vi "Handle Command.vi"(8 "error in (no error)":errorcluster, 9 "Data":variant, 10 "Command":string, 11 "VNA":refnum<class "VNA.lvclass">) -> (0 "error out":errorcluster, 1 "Processed Data":variant, 2 "Command":string, 3 "VNA out":refnum<class "VNA.lvclass">)   [LabVIEW 2016, in "VNA.lvclass"]
uses:
  VNA.lvclass
  VNA.lvclass/VNA.ctl
  <userlib>/LevyLab/Levylab Instruments/Instrument Types/VNA/Instrument.VNA.lvclass
  P:/users1/Dengyu/Agilent 87XX Series/Agilent 87XX Series.lvlib
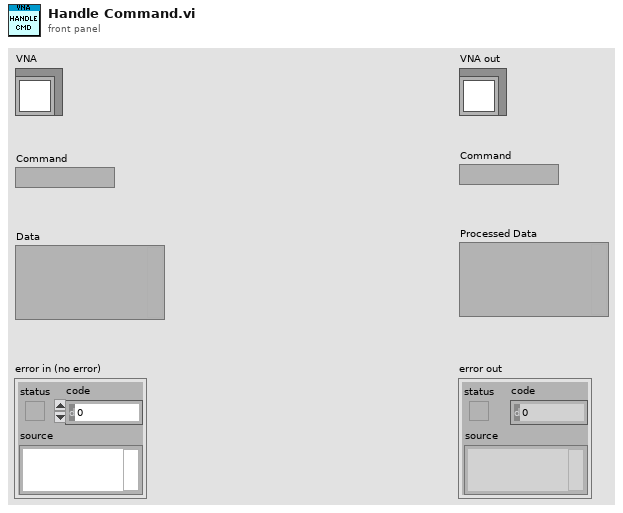
[diagram p1: front panel]
types:
  T1 = cluster{"Average?":enum16{"ON", "OFF"}, "Average Factor":i32}
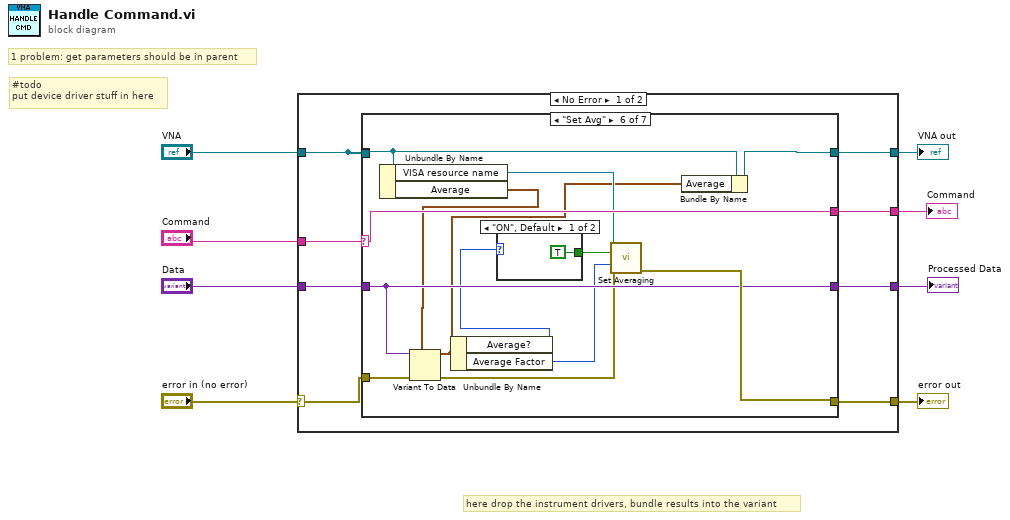
[diagram p0: block diagram]
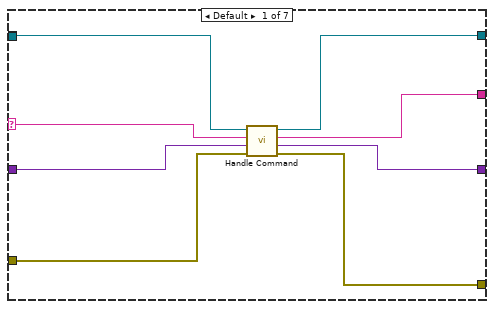
[diagram p2: hidden frame]
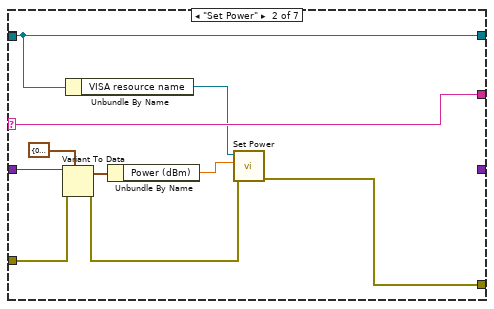
[diagram p3: hidden frame]
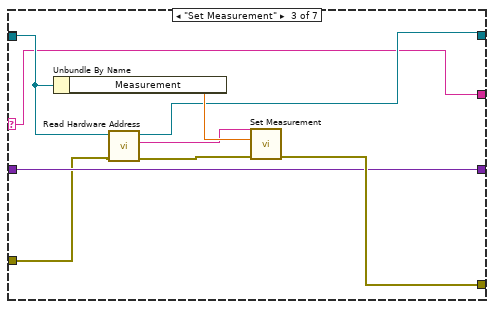
[diagram p4: hidden frame]
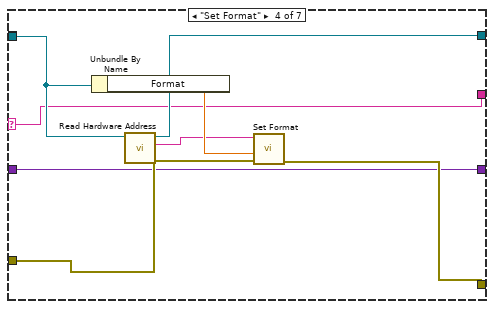
[diagram p5: hidden frame]
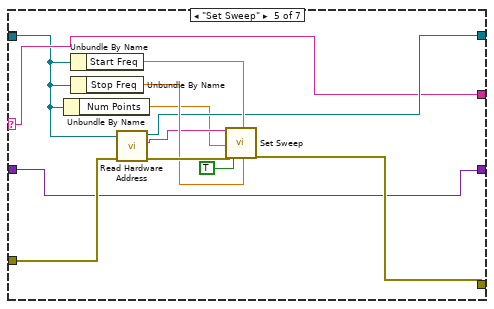
[diagram p6: hidden frame]
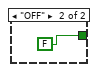
[diagram p7: hidden frame]
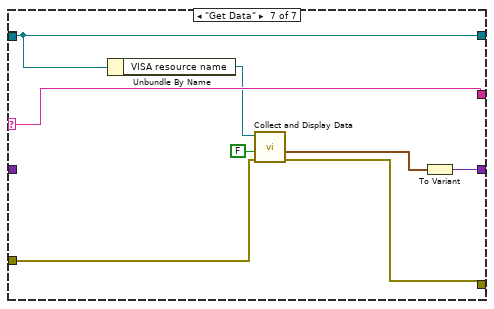
[diagram p8: hidden frame]
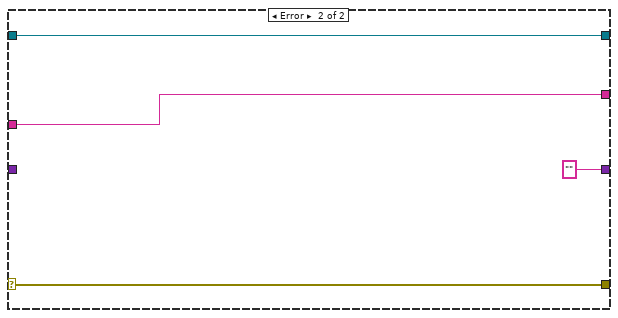
[diagram p9: hidden frame]
diagram:
  # "here drop the instrument drivers, bundle results into the variant"
  # "1 problem: get parameters should be in parent"
  # "#todo\nput device driver stuff in here"
  n1 = case shown="No Error" "error in (no error)" {
    selector: "error in (no error)" -> [w10 w91]
    tunnel: [w12 w91] -> w6
    tunnel: [w15 w90] -> w5
    tunnel: "VNA" -> [w9 w90]
    tunnel: "Command" -> [w16 w88]
    tunnel: [w14 "" ("String")] -> w3
    tunnel: "Data" -> [w13 _]
    tunnel: [w11 w88] -> w1
    frame No Error {
      n2 = case shown="\"Set Avg\"" w16 {
        selector: w16 -> [w24 w32 w37 w45 w56 w76 w84]
        tunnel: w9 -> [w21 w34 w39 _ w54 w66 w85]
        tunnel: [w18 w34 w38 w46 w57 w65 w85] -> w15
        tunnel: [w20 _ w36 w44 w55 w75 w82] -> w14
        tunnel: w10 -> [w22 w26 w35 w50 w63 w73 w87]
        tunnel: w13 -> [w23 w30 w36 w44 w55 w75 _]
        tunnel: [w19 w33 w42 w51 w64 w77 w86] -> w12
        tunnel: [w17 w32 w37 w45 w56 w76 w84] -> w11
        tunnel: w9 -> [_ _ _ w49 _ _ _]
        frame Default {
          n3 = call-parent "Handle Command.vi"("error in (no error)"=w22, "Data"=w23, "Command"=w24, "Instrument in"=w21) -> ("error out"=w19:errorcluster, "Processed Data"=w20:variant, "Command"=w17:string, "Instrument out"=w18:refnum<class "VNA.lvclass">)  [unwired: 4 in]
        }
        frame "Set Power" {
          n4 = Variant To Data(error in=w26, type=cluster{"Power (dBm)":dbl, "Channel":i32} {"Power (dBm)"=0.0, "Channel"=0} ("output cluster"), Variant=w30) -> (data=w28:cluster{"Power (dBm)":dbl, "Channel":i32}, error out=w25:errorcluster)
          n5 = Unbundle By Name(w34) -> ("VISA resource name"=w31:refnum<visa-resource-name>)
          n6 = Unbundle By Name(w28) -> ("Power (dBm)"=w27:dbl)
          n7 = call "Set Power.vi"("error in (no error)"=w25, "Power"=w27, "VISA resource name"=w31) -> ("error out"=w33:errorcluster)  [unwired: 7 in, 1 out]
        }
        frame "Set Measurement" {
          n8 = Unbundle By Name(w39) -> ("Measurement"=w41:dbl)
          n9 = call-dynamic "Read Hardware Address.vi"("error in (no error)"=w35, "Instrument in"=w39) -> ("error out"=w43:errorcluster, "Hardware Address"=w40:string, "Instrument out"=w38:refnum<class "VNA.lvclass">)  [unwired: 7 in]
          n10 = call "Set Measurement.vi"("error in (no error)"=w43, "measurement (0 : S11)"=w41, "VISA resource name"=w40) -> ("error out"=w42:errorcluster)  [unwired: 7 in, 1 out]
        }
        frame "Set Format" {
          n11 = Unbundle By Name(w49) -> ("Format"=w48:dbl)
          n12 = call-dynamic "Read Hardware Address.vi"("error in (no error)"=w50, "Instrument in"=w49) -> ("error out"=w52:errorcluster, "Hardware Address"=w47:string, "Instrument out"=w46:refnum<class "VNA.lvclass">)  [unwired: 7 in]
          n13 = call "Set Format.vi"("error in (no error)"=w52, "format (0 : log mag)"=w48, "VISA resource name"=w47) -> ("error out"=w51:errorcluster)  [unwired: 7 in, 1 out]
        }
        frame "Set Sweep" {
          n14 = Unbundle By Name(w54) -> ("Num Points"=w53:dbl)
          n15 = Unbundle By Name(w54) -> ("Start Freq"=w60:dbl)
          n16 = Unbundle By Name(w54) -> ("Stop Freq"=w59:dbl)
          n17 = call-dynamic "Read Hardware Address.vi"("error in (no error)"=w63, "Instrument in"=w54) -> ("error out"=w62:errorcluster, "Hardware Address"=w58:string, "Instrument out"=w57:refnum<class "VNA.lvclass">)  [unwired: 7 in]
          n18 = call "Set Sweep.vi"("VISA resource name"=w58, "num points"=w53, "error in (no error)"=w62, "t: start/stop  f: center/span"=TRUE, "start/center"=w60, "stop/span"=w59) -> ("error out"=w64:errorcluster)  [unwired: 12 in, 1 out]
        }
        frame "Set Avg" {
          n19 = Unbundle By Name(w66) -> ("VISA resource name"=w69:refnum<visa-resource-name>, "Average"=w68:T1)
          n20 = Variant To Data(error in=w73, type=w68, Variant=w75) -> (data=w67:T1, error out=w74:errorcluster)
          n21 = Unbundle By Name(w67) -> ("Average?"=w72:enum16{"ON", "OFF"}, "Average Factor"=w70:i32)
          n22 = case shown="\"ON\", Default" w72 {
            tunnel: [TRUE ("average (F : off)") FALSE ("average (F : off)")] -> w71
            frame "ON", Default {
            }
            frame "OFF" {
            }
          }
          n23 = call "Set Averaging.vi"("VISA resource name"=w69, "average (F : off)"=w71, "average factor (16)"=w70, "error in (no error)"=w74) -> ("error out"=w77:errorcluster)  [unwired: 10 in, 1 out]
          n24 = Bundle By Name(cluster=w66, "Average"=w67) -> (w65:refnum<class "VNA.lvclass">)
        }
        frame "Get Data" {
          n25 = Unbundle By Name(w85) -> ("VISA resource name"=w80:refnum<visa-resource-name>)
          n26 = call "Collect and Display Data.vi"("error in (no error)"=w87, "save to file"=FALSE, "VISA resource name"=w80) -> ("error out"=w86:errorcluster, "data values"=w83:cluster{"real / stim":dbl, "imag / resp":sgl}[])  [unwired: 5 in, 2 out]
          n27 = To Variant(anything=w83) -> (Variant=w82:variant)
        }
      }
    }
    frame Error {
    }
  }
  "error out" <- w6
  "VNA out" <- w5
  "Command" <- w1
  "Processed Data" <- w3
